vi "plate_zero_v2.vi"(8 "error in":errorcluster, 10 "DO array":bool[](array[boolean]), 11 "tasks":T1) -> (0 "error out":errorcluster)   [LabVIEW 2013]
uses:
  <vilib>/DAQmx/write.llb/DAQmx Write (Digital 1D Bool NChan 1Samp 1Line).vi
  <vilib>/DAQmx/read.llb/DAQmx Read (Digital 1D Bool NChan 1Samp 1Line).vi
  <vilib>/DAQmx/configure/timing.llb/DAQmx Timing (Implicit).vi
  <vilib>/DAQmx/miscellaneous.llb/DAQmx Fill In Error Info.vi
  <resource>/objmgr/daqmx.rc
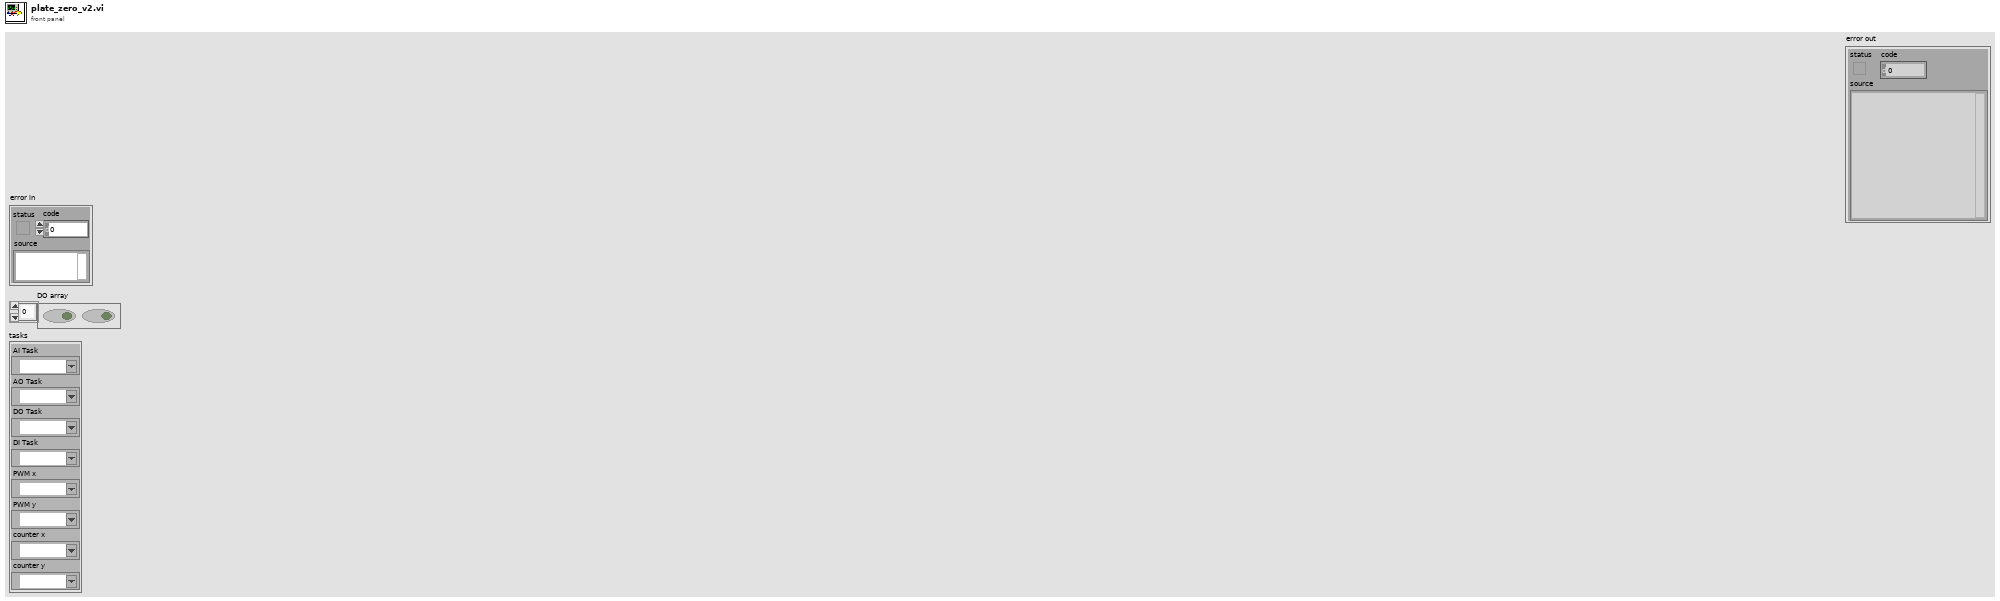
[diagram p1: front panel]
types:
  T1 = cluster{"AI Task":refnum<k21>, "AO Task":refnum<k21>, "DO Task":refnum<k21>, "DI Task":refnum<k21>, "PWM x":refnum<k21>, "PWM y":refnum<k21>, "counter x":refnum<k21>, "counter y":refnum<k21>}
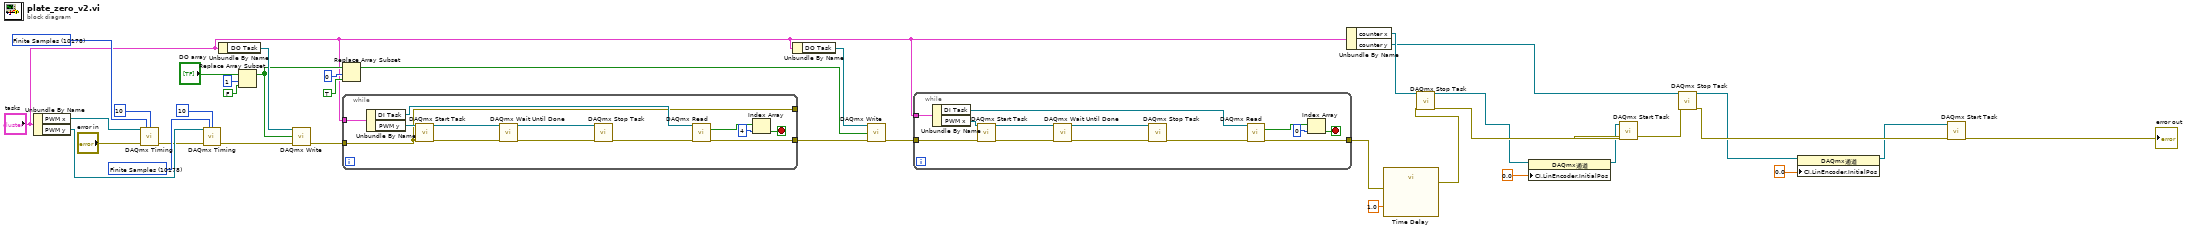
[diagram p0: block diagram]
diagram:
  w34 = 10178 items=["Finite Samples"=10178, "Continuous Samples"=10123, "Hardware Timed Single Point"=12522] ("sample mode")
  w36 = 10178 items=["Finite Samples"=10178, "Continuous Samples"=10123, "Hardware Timed Single Point"=12522] ("sample mode")
  n1 = Unbundle By Name("tasks") -> ("PWM x"=w37:refnum<k21>, "PWM y"=w32:refnum<k21>)
  n2 = call-poly <vilib>:"DAQmx Timing.vi"("task/channels in"=w37, "sample mode"=w36, "samples per channel"=10, "error in"="error in") -> ("error out"=w31:errorcluster)  [unwired: 10 in, 1 out]
  n3 = call-poly <vilib>:"DAQmx Timing.vi"("task/channels in"=w32, "sample mode"=w34, "samples per channel"=10, "error in"=w31) -> ("error out"=w19:errorcluster)  [unwired: 10 in, 1 out]
  n4 = Unbundle By Name("tasks") -> ("DO Task"=w27:refnum<k21>)
  n5 = Replace Array Subset(array="DO array", new element=FALSE ("new element/subarray"), index=1) -> (w24:bool[])
  n6 = call-poly <vilib>:"DAQmx Write.vi"("task/channels in"=w27, "data"=w24, "error in"=w19) -> ("error out"=w30:errorcluster)  [unwired: 10 in, 2 out]
  n7 = Replace Array Subset "Replace Array Subset"(array=w24, new element=TRUE ("new element/subarray"), index=0) -> (w17:bool[])
  n8 = while {
    tunnel: [w38] -> _
    tunnel: "tasks" -> [w50]
    tunnel: [w39] -> w18
    tunnel: w30 -> [w38]
    stop <- w46 stop-if-true
    n9 = Unbundle By Name(w50) -> ("DI Task"=w49:refnum<k21>, "PWM y"=w45:refnum<k21>)
    n10 = call <vilib>:"DAQmx Start Task.vi"("task/channels in"=w45, "error in"=w38) -> ("task out"=w43:refnum<k21>, "error out"=w44:errorcluster)  [unwired: 12 in]
    n11 = call <vilib>:"DAQmx Wait Until Done.vi"("task/channels in"=w43, "error in"=w44) -> ("task out"=w40:refnum<k21>, "error out"=w42:errorcluster)  [unwired: 12 in]
    n12 = call <vilib>:"DAQmx Stop Task.vi"("task/channels in"=w40, "error in"=w42) -> ("error out"=w41:errorcluster)  [unwired: 12 in, 1 out]
    n13 = call-poly <vilib>:"DAQmx Read.vi"("task/channels in"=w49, "error in"=w41) -> ("data"=w48:bool[], "error out"=w39:errorcluster)  [unwired: 11 in, 1 out]
    n14 = Index Array(array=w48, index=4) -> (element=w46:bool)
  }
  n15 = Unbundle By Name("tasks") -> ("DO Task"=w25:refnum<k21>)
  n16 = call-poly <vilib>:"DAQmx Write.vi"("task/channels in"=w25, "data"=w17, "error in"=w18) -> ("error out"=w26:errorcluster)  [unwired: 10 in, 2 out]
  n17 = while {
    tunnel: "tasks" -> [w63]
    tunnel: [w52] -> w15
    tunnel: w26 -> [w51]
    stop <- w59 stop-if-true
    n18 = Unbundle By Name(w63) -> ("DI Task"=w62:refnum<k21>, "PWM x"=w58:refnum<k21>)
    n19 = call <vilib>:"DAQmx Start Task.vi"("task/channels in"=w58, "error in"=w51) -> ("task out"=w56:refnum<k21>, "error out"=w57:errorcluster)  [unwired: 12 in]
    n20 = call <vilib>:"DAQmx Wait Until Done.vi"("task/channels in"=w56, "error in"=w57) -> ("task out"=w53:refnum<k21>, "error out"=w55:errorcluster)  [unwired: 12 in]
    n21 = call <vilib>:"DAQmx Stop Task.vi"("task/channels in"=w53, "error in"=w55) -> ("error out"=w54:errorcluster)  [unwired: 12 in, 1 out]
    n22 = call-poly <vilib>:"DAQmx Read.vi"("task/channels in"=w62, "error in"=w54) -> ("data"=w61:bool[], "error out"=w52:errorcluster)  [unwired: 11 in, 1 out]
    n23 = Index Array(array=w61, index=0) -> (element=w59:bool)
  }
  n24 = Unbundle By Name("tasks") -> ("counter x"=w14:refnum<k21>, "counter y"=w12:refnum<k21>)
  n25 = call "Time Delay"("error in (no error)"=w15, "Delay Time (s)"=1.0) -> ("error out"=w2:errorcluster)  [unwired: 9 in]
  n26 = call <vilib>:"DAQmx Stop Task.vi"("task/channels in"=w14, "error in"=w2) -> ("task out"=w9:refnum<k21>, "error out"=w11:errorcluster)  [unwired: 12 in]
  n27 = property class="DAQmx通道"(reference=w9, "CI.LinEncoder.InitialPos"=0.0) -> (reference out=w7:refnum<k21>)  [unwired: 1 in, 1 out]
  n28 = call <vilib>:"DAQmx Start Task.vi"("task/channels in"=w7, "error in"=w11) -> ("error out"=w13:errorcluster)  [unwired: 12 in, 1 out]
  n29 = call <vilib>:"DAQmx Stop Task.vi"("task/channels in"=w12, "error in"=w13) -> ("task out"=w6:refnum<k21>, "error out"=w10:errorcluster)  [unwired: 12 in]
  n30 = property class="DAQmx通道"(reference=w6, "CI.LinEncoder.InitialPos"=0.0) -> (reference out=w5:refnum<k21>)  [unwired: 1 in, 1 out]
  n31 = call <vilib>:"DAQmx Start Task.vi"("task/channels in"=w5, "error in"=w10) -> ("error out"=→"error out":errorcluster)  [unwired: 12 in, 1 out]
